vi "Main MATE GUI.vi"() -> ()   [LabVIEW 2012]
doc: "This vi connects to a Joystick via Microsoft's Human Interface Devices and passes the necessary controls to the \"Remote\" variables \nSee Block Diagram:\n1. Quarry about available joystick\n2. Search for the joystick with the specified device\n3. If no match is found, then pass an error, then try and initialize the device\n4. Use a timed wile loop to save recourse, just looping and poling the joystick data is capable of high loop speeds\n5. Get Joystick sensor data\n6. Set the Trigger enable condition and pass along the XY data\n7. Normalize the values and use a running average to smooth out the control\n8. Apply expo weight for less sensitive control and zero out dead stick offset \n9. Set XY data\n10. XY plot is data binding to network variable for the XY plot on HUD from the Remote tab\n11. Use a stop button titled \"stop?\" so that the LabVIEW script can stop the vi\n12. Close the Joystick connection\n-Ruffin White\n-Kyle Green"
uses:
  Support/Teleop command.ctl
  <vilib>/Platform/TimedLoop/XDataNode/timing_clust.ctl
  <vilib>/Platform/TimedLoop/XDataNode/nitl_modes.ctl
  <vilib>/Platform/TimedLoop/XDataNode/wakeup.ctl
  Support/Host globals (robot acquires video).vi
  <vilib>/Platform/TimedLoop/XDataNode/XDataNode.xnode
  ROV Host.lvclass
  <vilib>/Platform/TimedLoop/XDataNode/XDNodeRunTimeDep.lvlib
panel:
  out "Side View":picture
  out "Top View":picture
  out "Error":bool
  in  "Telemetry":T1(tab)
  in  "ROV IP address":string="XXX.XXX.XXX.XXX"
  out "Teleop command":T2
  out "Listed Devices":T3(array[cluster])
  in  "Device Name":string="Controller (XBOX 360 For Windows)" caption="Give the exact \"divice name\" string of the joypad you would like to use."
  in  "Expo":dbl(slide)=1.0 scale=0.0..10.0
  out "Comunication Error":errorcluster
  out "Joypad Error":errorcluster
  out "error out":errorcluster
  in  "Error in":errorcluster
  in  "Robot Mode:":T4(ring)
  in  "Stop":bool
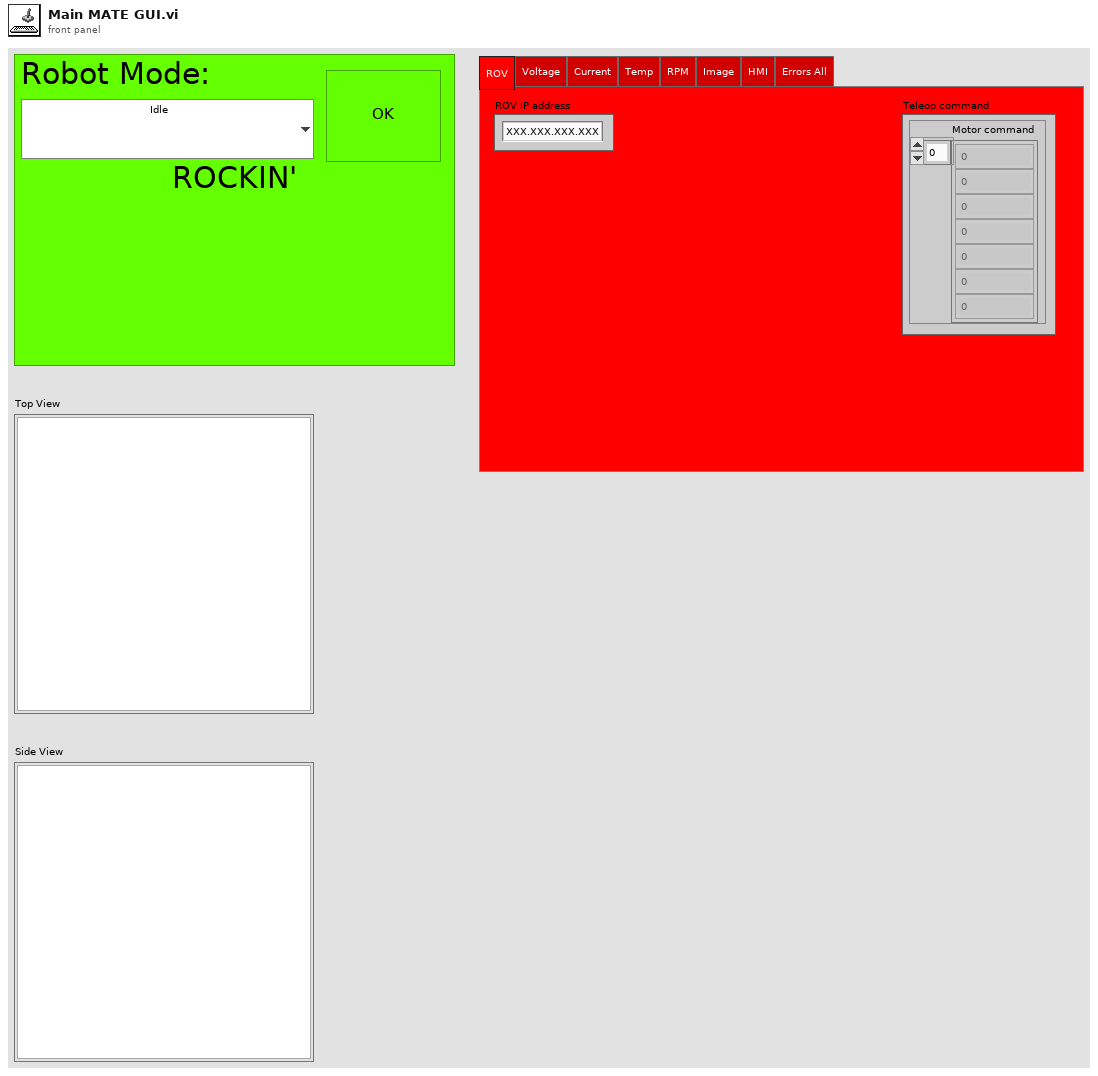
[diagram p1: front panel]
types:
  T1 = enum32{"ROV", "Voltage", "Current", "Temp", "RPM", "Image", "HMI", "Errors All"}
  T2 = typedef "Teleop command.ctl" = cluster{"Motor command":dbl[]}
  T3 = cluster{"axes total":u32, "buttons total":u32, "pov total":u32, "device name":string}[]
  T4 = enum16{"Idle", "Calibrate", "Teleoperation", "Abort"}
  T5 = typedef "XDNodeRunTimeDep.lvlib/timing_clust.ctl" = cluster{"Expected End [f-1]":u64, "Actual End [f-1]":u64, "Finished Late? [f-1]":bool, "Expected End [i-1]":u64, "Actual End [i-1]":u64, "Finished Late? [i-1]":bool, "Expected Start [i]":u64, "Actual Start [i]":u64, "Expected Start [f]":u64, "Actual Start [f]":u64, "Source Name":string, "Structure Name":string, "Period":i64, "Deadline":i64, "Offset":i64, "Start":i64, "Priority":i32, "Timeout":i32, "Mode":T6, "Wakeup Reason":T7, "Error":errorcluster, "Source Type":string, "Secondary Source Type":string, "Global End Time":u64, "Global Start Time":u64, "Frame Duration":u64, "Iteration Duration":u64, "Assigned CPU":i32, "I/O Scan Engine Mode":u32}
  T6 = typedef "XDNodeRunTimeDep.lvlib/nitl_modes.ctl" = enum32{"No Change", "Process missed periods, maintain original phase", "Discard missed periods, maintain original phase", "Process missed periods, ignore original phase", "Discard missed periods, ignore original phase"}
  T7 = typedef "XDNodeRunTimeDep.lvlib/wakeup.ctl" = enum32{"Normal", "Aborted", "Asynchronous wakeup", "Timing source error", "Timed loop error", "Timeout"}
  T8 = typedef "LVBoundsTypeDef.ctl" = cluster{"Width":u32, "Height":u32}
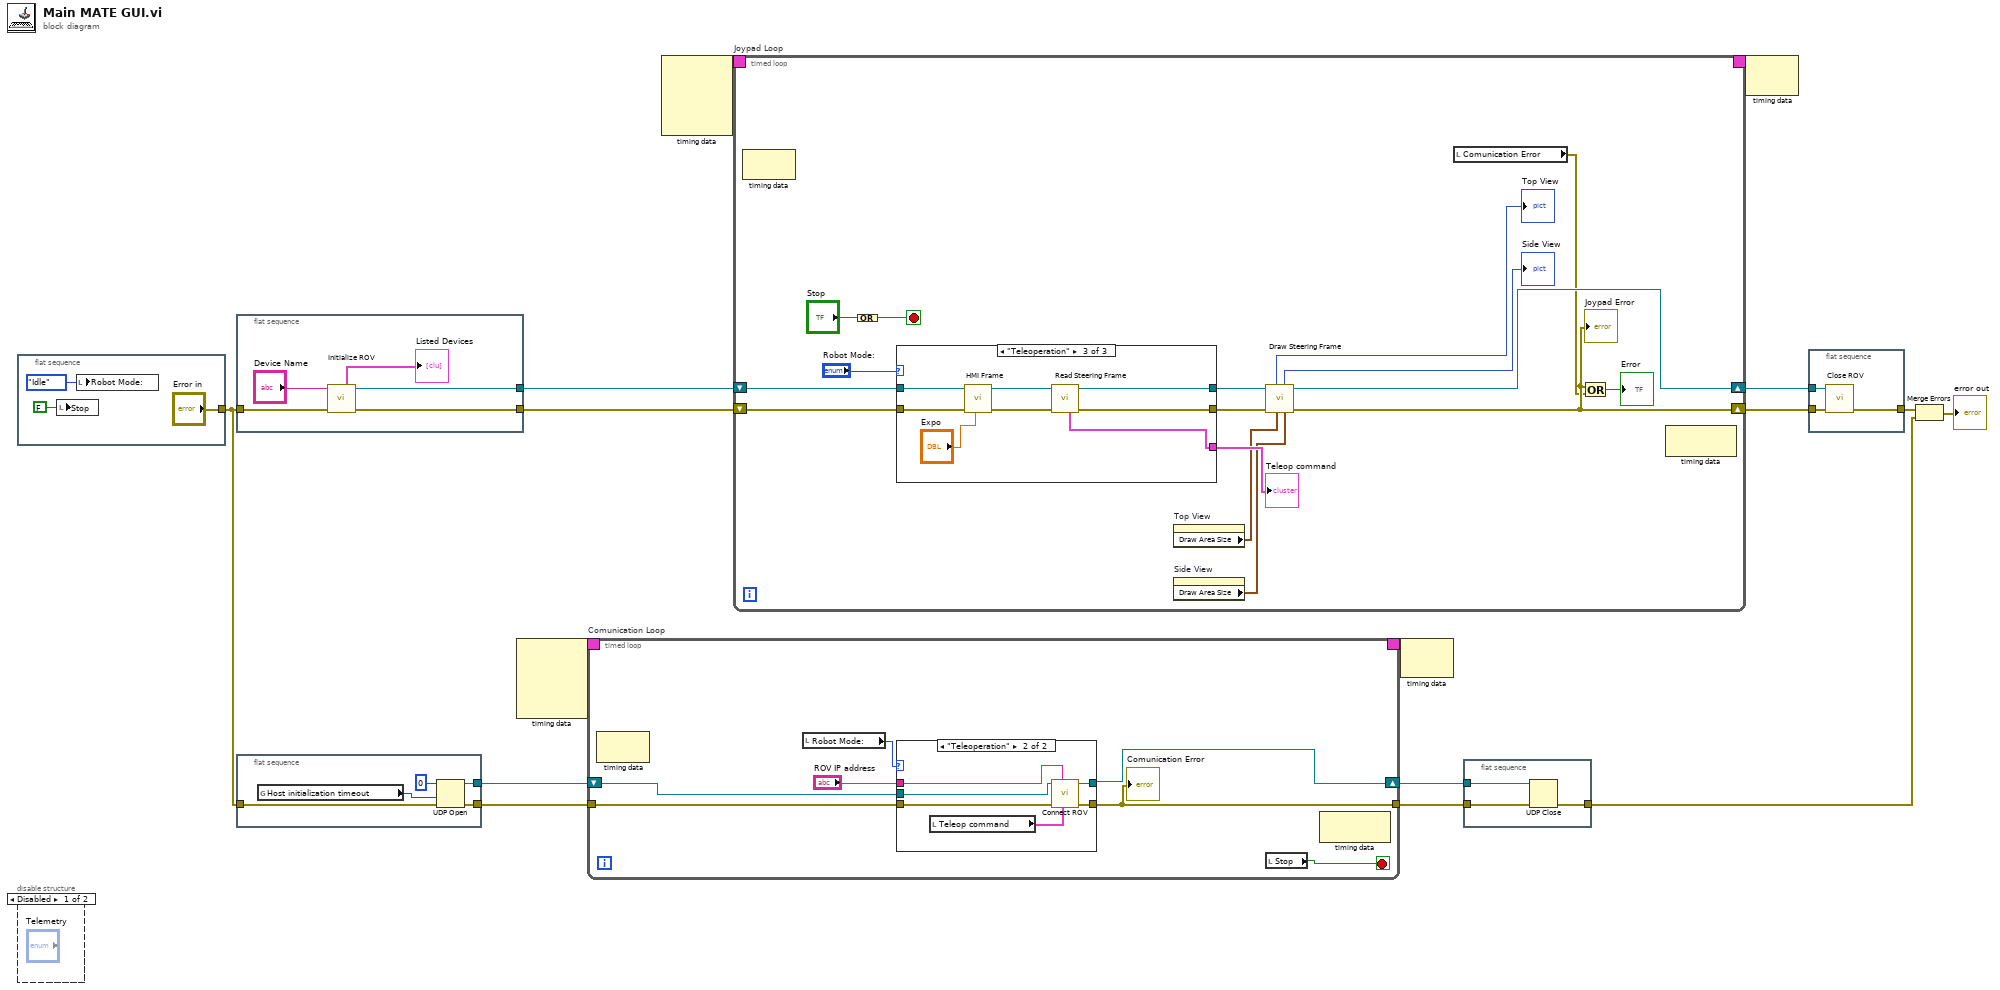
[diagram p0: block diagram]
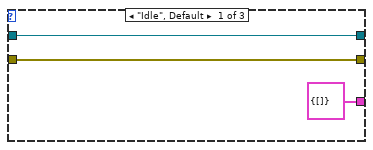
[diagram p4: hidden frame]
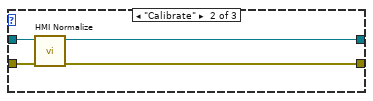
[diagram p5: hidden frame]
diagram:
  n1 = flat-sequence {
    tunnel: ["Error in"] -> w10
    frame #0 {
      n2 = local write "Stop"(FALSE ("Stop")) -> ()
      n3 = local write "Robot Mode:"(T4."Idle" ("Robot Mode:")) -> ()
    }
  }
  n4 = disable-structure shown="Disabled" {
    frame Disabled {
    }
    frame Enabled {
    }
  }
  n5 = flat-sequence {
    tunnel: [w24] -> w9
    tunnel: [w21] -> w14
    tunnel: w10 -> [w20]
    frame #0 {
      n6 = call "Initialize ROV.vi"("error in (no error)"=w20, "Device Name"="Device Name") -> ("error out"=w24:errorcluster, "ROV Host.lvclass"=w21:refnum<class "ROV Host.lvclass">, "Listed Devices"=→"Listed Devices":T3)  [unwired: 7 in]
    }
  }
  n7 = flat-sequence {
    tunnel: w10 -> [w27]
    tunnel: [w26] -> w8
    tunnel: [w25] -> w5
    frame #0 {
      n8 = global read "Host globals (robot acquires video).vi" "Host initialization timeout"() -> (w29:i32)
      n9 = UDP Open(8:w27, 9:w29, 11:u16 0 ("port")) -> (port=w25:refnum<k16>, 0:w26:errorcluster)  [unwired: 2 in, 1 out]
    }
  }
  n10 = node-c288() -> (w12:T5)  [unwired: 4 in]
  n11 = timed-loop "Comunication Loop" {
    timing: w12 -> [_]
    timing-out: [_] -> w11
    shift-right: [w31] -> w6
    shift-left: w5 -> [w32]
    tunnel: w8 -> [w34]
    tunnel: [w33] -> w7
    stop <- w35 stop-if-true
    n12 = node-c288() -> ()  [unwired: 1 in, 1 out]
    n13 = local read "Robot Mode:"() -> (w36:T4)
    n14 = case shown="\"Teleoperation\"" w36 {
      tunnel: w34 -> [w38 w44]
      tunnel: [w38 w43] -> w33
      tunnel: w32 -> [w37 w42]
      tunnel: [w37 w41] -> w31
      tunnel: "ROV IP address" -> [_ w40]
      frame "Idle", Default {
      }
      frame "Teleoperation" {
        n15 = local read "Teleop command"() -> (w39:T2)
        n16 = call "Connect ROV.vi"("Teleop command"=w39, "IP address"=w40, "error in (no error)"=w44, "connection ID"=w42) -> ("error out"=w43:errorcluster, "connection ID out"=w41:refnum<k16>)  [unwired: 6 in]
      }
    }
    "Comunication Error" <- w33
    n17 = local read "Stop"() -> (w35:bool)
    n18 = node-c288() -> ()  [unwired: 1 in, 1 out]
  }
  n19 = node-c288() -> (w16:T5)  [unwired: 4 in]
  n20 = timed-loop "Joypad Loop" {
    timing: w16 -> [_]
    timing-out: [_] -> w15
    shift-right: [w53] -> w13
    shift-left: w14 -> [w55]
    shift-right: [w49] -> w2
    shift-left: w9 -> [w60]
    stop <- w62 stop-if-true
    n21 = node-c288() -> ()  [unwired: 1 in, 1 out]
    n22 = Compound Arithmetic op=OR("Stop") -> (w62:bool)
    n23 = case shown="\"Teleoperation\"" "Robot Mode:" {
      tunnel: w60 -> [w65 w68 w77]
      tunnel: [w65 w69 w74] -> w59
      tunnel: w55 -> [w64 w67 w76]
      tunnel: [w64 w66 w71] -> w54
      tunnel: [T2 {"Motor command"=[]} ("Teleop command") _ w70] -> w52
      frame "Idle", Default {
      }
      frame "Calibrate" {
        n24 = call "HMI Normalize.vi"("error in (no error)"=w68, "ROV in"=w67) -> ("error out"=w69:errorcluster, "ROV out"=w66:refnum<class "ROV Host.lvclass">)  [unwired: 8 in]
      }
      frame "Teleoperation" {
        n25 = call "HMI Frame.vi"("Expo"="Expo", "error in (no error)"=w77, "ROV in"=w76) -> ("error out"=w73:errorcluster, "ROV out"=w72:refnum<class "ROV Host.lvclass">)  [unwired: 7 in]
        n26 = call "Read Steering Frame.vi"("error in (no error)"=w73, "ROV in"=w72) -> ("error out"=w74:errorcluster, "ROV out"=w71:refnum<class "ROV Host.lvclass">, "Teleop command"=w70:T2)  [unwired: 7 in]
      }
    }
    "Teleop command" <- w52
    n27 = property on="Top View" class="Pict"() -> ("Draw Area Size"=w51:T8)  [unwired: 2 in, 2 out]
    n28 = property on="Side View" class="Pict"() -> ("Draw Area Size"=w50:T8)  [unwired: 2 in, 2 out]
    n29 = call "Draw Steering Frame.vi"("Side View Draw Area Size 2"=w50, "Top View Draw Area Size"=w51, "error in (no error)"=w59, "ROV in"=w54) -> ("error out"=w49:errorcluster, "ROV out"=w53:refnum<class "ROV Host.lvclass">, "Side View"=→"Side View":picture, "Top View"=→"Top View":picture)  [unwired: 4 in]
    "Joypad Error" <- w49
    n30 = local read "Comunication Error"() -> (w48:errorcluster)
    n31 = Compound Arithmetic op=OR(w49, w48) -> (→"Error":bool)
    n32 = node-c288() -> ()  [unwired: 1 in, 1 out]
  }
  n33 = node-c288(w11) -> ()  [unwired: 1 out]
  n34 = flat-sequence {
    tunnel: w7 -> [w82]
    tunnel: [w81] -> w4
    tunnel: w6 -> [w80]
    frame #0 {
      n35 = UDP Close(connection ID=w80, 8:w82) -> (error out=w81:errorcluster)  [unwired: 1 out]
    }
  }
  n36 = node-c288(w15) -> ()  [unwired: 1 out]
  n37 = flat-sequence {
    tunnel: w13 -> [w85]
    tunnel: w2 -> [w84]
    tunnel: [w83] -> w3
    frame #0 {
      n38 = call "Close ROV.vi"("error in (no error)"=w84, "ROV in"=w85) -> ("error out"=w83:errorcluster)  [unwired: 9 in]
    }
  }
  n39 = Merge Errors(w3, w4) -> (→"error out":errorcluster)
